vi "Execute.vi"(8 "error in (no error)":errorcluster, 11 "Node in":refnum<class "bt_Log.lvclass">) -> (0 "error out":errorcluster, 1 "Status":T1, 3 "Node out":refnum<class "bt_Log.lvclass">)   [LabVIEW 2021, in "BT.lvlib" / "bt_Log.lvclass"]
uses:
  bt_Log.lvclass
  abs_Node/Status.ctl
  bt_Log.lvclass/bt_Log.ctl
  <vilib>/TSA/Abstract Data Classes/Abs_Types/String/Static Read.vi
  Properties/Read EventLog.vi
  Properties/Read Message.vi
  Properties/Write EventLog.vi
  Properties/Write Message.vi
  <vilib>/TSA/Event Log/abs_EventLog/abs_EventLog.lvclass
  <vilib>/TSA/Abstract Data Classes/Abs_Types/String/Abs_String.lvclass
  abs_Node/bt_Node.lvclass
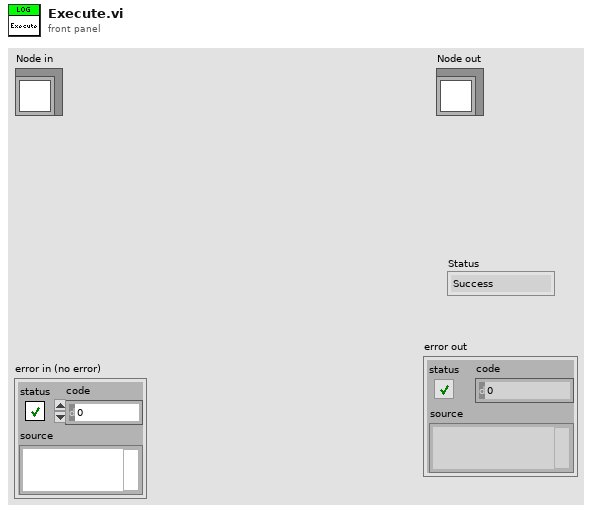
[diagram p1: front panel]
types:
  T1 = typedef "BT.lvlib/bt_Node.lvclass/Status.ctl" = enum16{"Success", "Failure", "Running"}
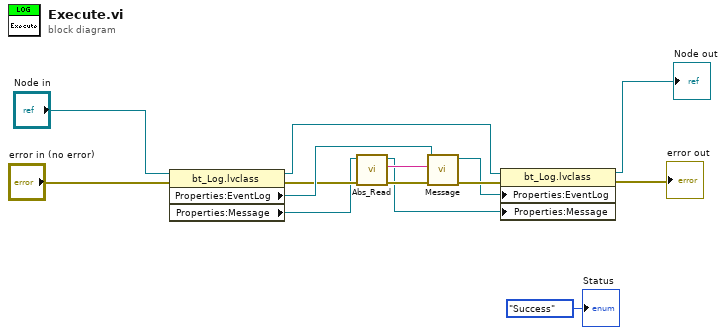
[diagram p0: block diagram]
diagram:
  n1 = property class="bt_Log.lvclass"(reference="Node in", error in="error in (no error)") -> (reference out=w7:refnum<class "bt_Log.lvclass">, error out=w3:errorcluster, "Properties:EventLog"=w11:refnum<class "abs_EventLog.lvclass">, "Properties:Message"=w2:refnum<class "Abs_String.lvclass">)
  n2 = call-poly <vilib>:"Abs_Read.vi"("error in (no error)"=w3, "Abs_String in"=w2) -> ("error out"=w5:errorcluster, "String"=w4:string, "Abs_String out"=w1:refnum<class "Abs_String.lvclass">)  [unwired: 7 in]
  n3 = call-dynamic "Message.vi"("error in (no error)"=w5, "Message"=w4, "abs_EventLog in"=w11) -> ("error out"=w10:errorcluster, "abs_EventLog out"=w9:refnum<class "abs_EventLog.lvclass">)  [unwired: 7 in]
  n4 = property class="bt_Log.lvclass"(reference=w7, error in=w10, "Properties:EventLog"=w9, "Properties:Message"=w1) -> (reference out=→"Node out":refnum<class "bt_Log.lvclass">, error out=→"error out":errorcluster)
  "Status" <- Status."Success" ("Status")
